vi "host_for_Tx_and_Rx_with scope_scope_cal_file_gen.vi"() -> ()   [LabVIEW 2021]
uses:
  <vilib>/userdefined/High Color/nirio_resource_hc.ctl
  use with scope/states_for scope.ctl
  classes/5785_2_x_1600MHz/5785_2_x_1600MHz.lvclass
  C:/Users/PXIe8108_Demo/Documents/CHAIM DATA/chaim/5785_sync_for_elbit/tx_pulse/pulse Tx Folder_lv_21/EMEA_ADG_EW_Multi_Emitter_Scenarios/classes/device_type/device_type.lvclass
  CTL/user config.ctl
  <instrlib>/niScope/Controls/niScope vertical coupling.ctl
  <instrlib>/niScope/Controls/niScope timestamp type.ctl
  <vilib>/Analysis/1siggen.llb/Ramp Pattern by Delta.vi
  <instrlib>/niScope/Configure/Trigger/niScope Configure Trigger Edge.vi
  <instrlib>/niScope/Acquire/Fetch/niScope Multi Fetch WDT.vi
  <vilib>/Analysis/NI_AALBase.lvlib
  classes/device_type/device_type.lvclass
panel:
  out "run number":i32
  in  "number of runs for cal":dbl=15.0 format="%#_13g"
  in  "read file":bool
  in  "save file":bool=TRUE
  in  "file path":path=path "C:/Users/PXIe8108_Demo/Documents/CHAIM DATA/chaim/5785_sync_for_elbit/tx_pulse/pulse Tx Folder_lv_21/EMEA_ADG_EW_Multi_Emitter_Scenarios/data/scope_cal_file.tdms"
  out "state":T1
  in  "cal":bool=TRUE
  in  "cal mode":bool=TRUE
  out "delta phase(deg)":cluster{"freqency":dbl[], "Array":dbl[]}[](graph)
  out "delta amp (dB)":cluster{"Array":dbl[], "Array":dbl[]}[](graph)
  in  "Channel Name":string="0,3"
  in  "Resource Name":refnum<k15>="scope1" caption="Resource Name(s)"
  in  "pulse amplitude (dB)":dbl=-40.0 format="%#_13g"
  in  "pulse duration (s)":dbl=0.0002 format="%#_13p"
  in  "frequncy comb":cluster{"start":dbl, "end":dbl, "delta":dbl}={"start"=5000000.0, "end"=300000000.0, "delta"=500000.0} {"delta" format="%#_6p"; "end" format="%#_6p"; "start" format="%#_6p"}
  in  "devicess":T2[](array[typedef])=["5785_00", "5785_01", "5785_02"]
  # "5785 system alignment scope cal"
  # "RF setup"
  # "Cal Data"
  # "HW setup"
  # "scope mapping:\nchannel 0 => 5785_02 _0 \nchannel 1 => 5785_01 _0 \nchannel 2 => 5785_01 _1 \nchannel 3 => 5785_00 _1"
  # "Cal test"
  # "SW setup"
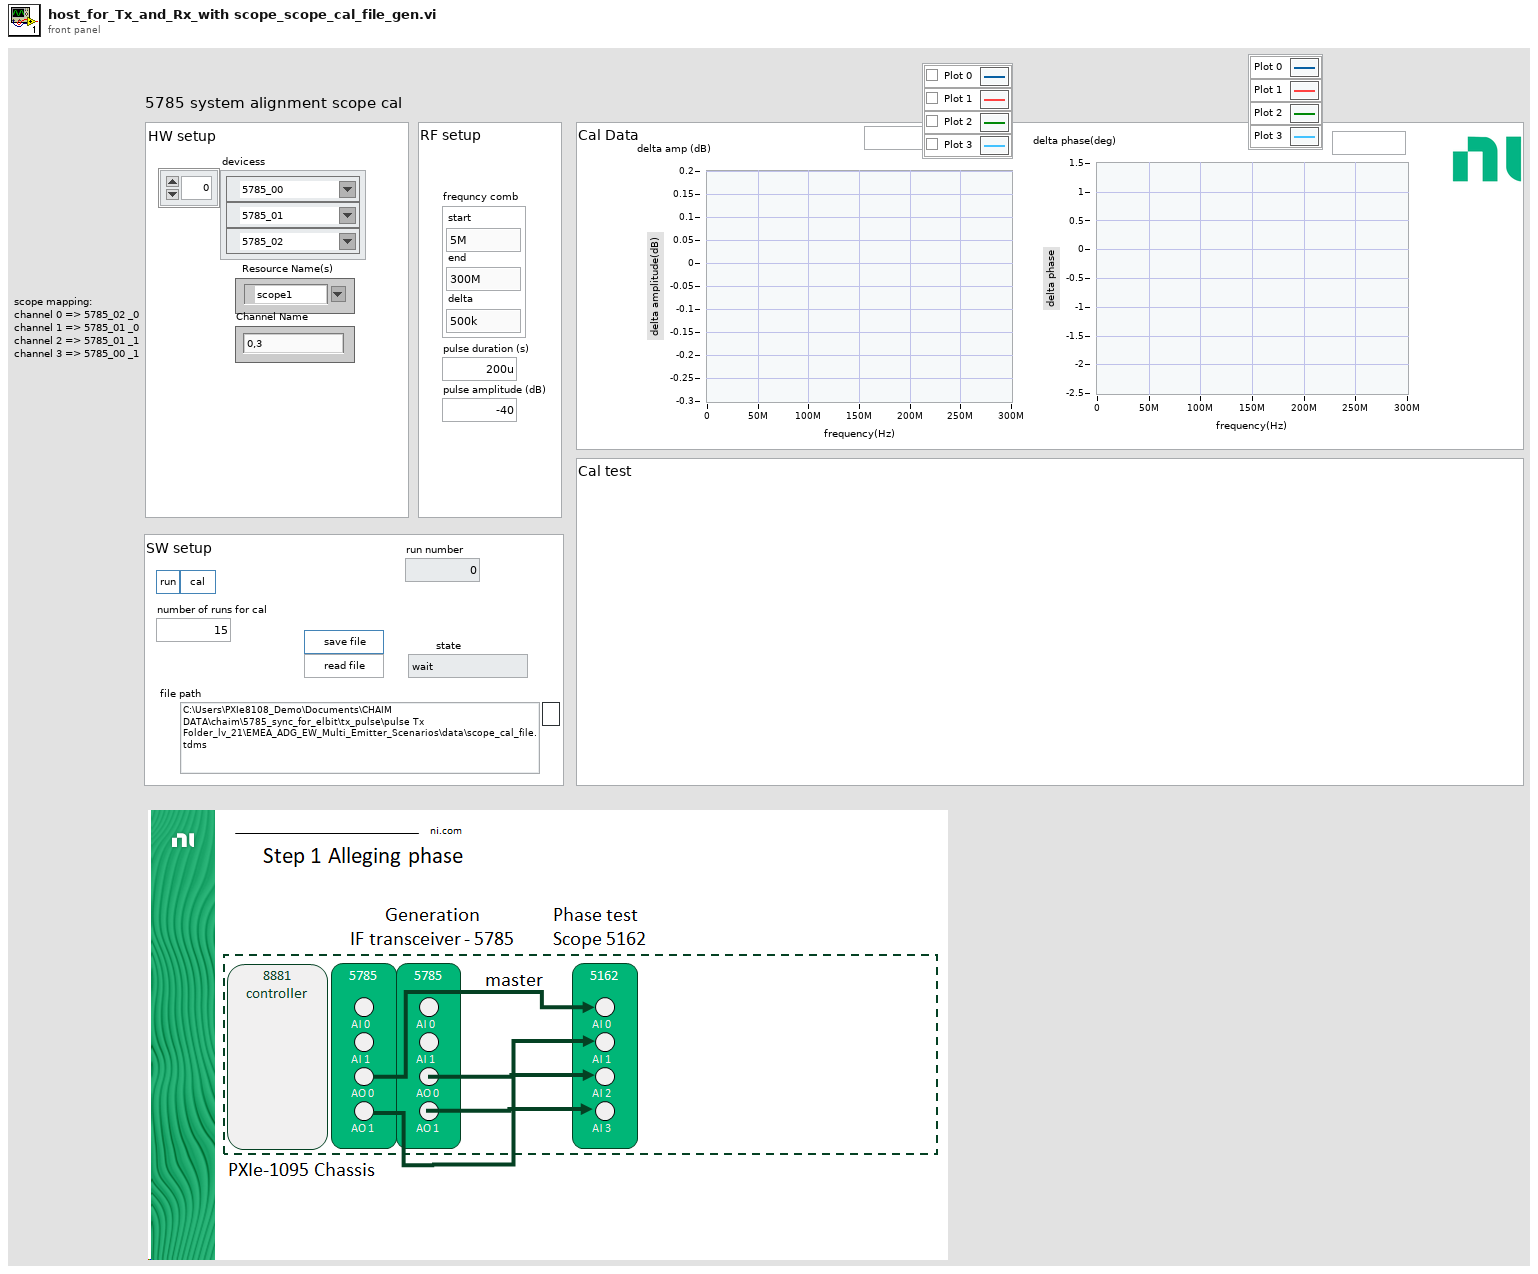
[diagram p1: front panel]
types:
  T1 = typedef "states_for scope.ctl" = enum16{"wait", "update ME config", "gen secenario", "INI ME", "INI scope", "trig", "close ME", "run mesearment", "save cal data", "get file data", "gen PDW file", "keep the data", "reset memory data", "prime the fifo"}
  T2 = typedef "nirio_resource_hc.ctl" = tag
  T3 = cluster{"freqency":dbl[], "phase":dbl[], "amp":dbl[]}[]
  T4 = cluster{"freqency":dbl[], "phase":dbl[], "amp":dbl[]}
  T5 = typedef "user config.ctl" = cluster{"vst_device":refnum<k15>[], "RF gain ":dbl, "buffer size":u32, "center frequency (Hz) ":dbl, "P2P sample rate":dbl, "mode":enum16{"USRP - 180MHz", "5785 - 2*180MHz", "5785 - 3.2GHz", "P2P - VST"}, "devicess":T2[], "gen for df":bool, "Rx settings":cluster{"min PW         ":dbl, "max gap        ":dbl, "detection bar":dbl, "peak detect                        ":bool}, "use arb files":bool}
  T6 = enum16{"open", "open or create", "create or replace", "create", "open (read-only)"}
  T7 = typedef "niScope vertical coupling.ctl" = i32
  T8 = typedef "PDW_lv2.ctl" = cluster{"t start":dbl, "frequency (Hz)":dbl, "duration (sec)":dbl, "mod type":T9, "mod depth":dbl, "phase (rad)":dbl[], "amp (lin)":dbl[]}
  T9 = typedef "mode_type.ctl" = enum8{"CW", "from memory 1", "NC - cw", "LFM", "BPSK", "QPSK"}
  T10 = typedef "niScope timestamp type.ctl" = i32
  T11 = cluster{"frequncy":dbl, "d amp":dbl, "d phase":dbl}[]
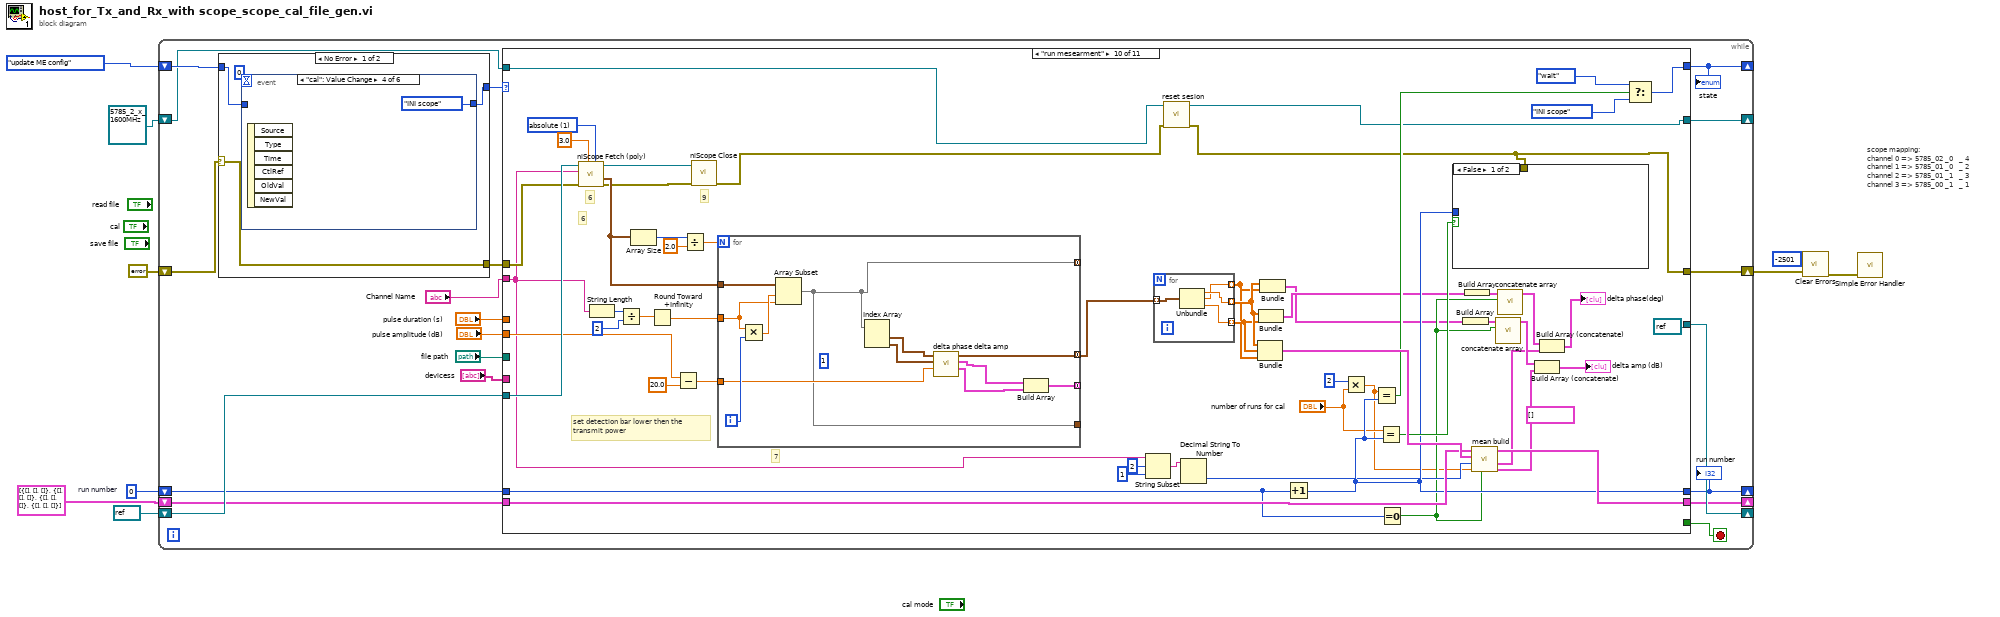
[diagram p0: block diagram]
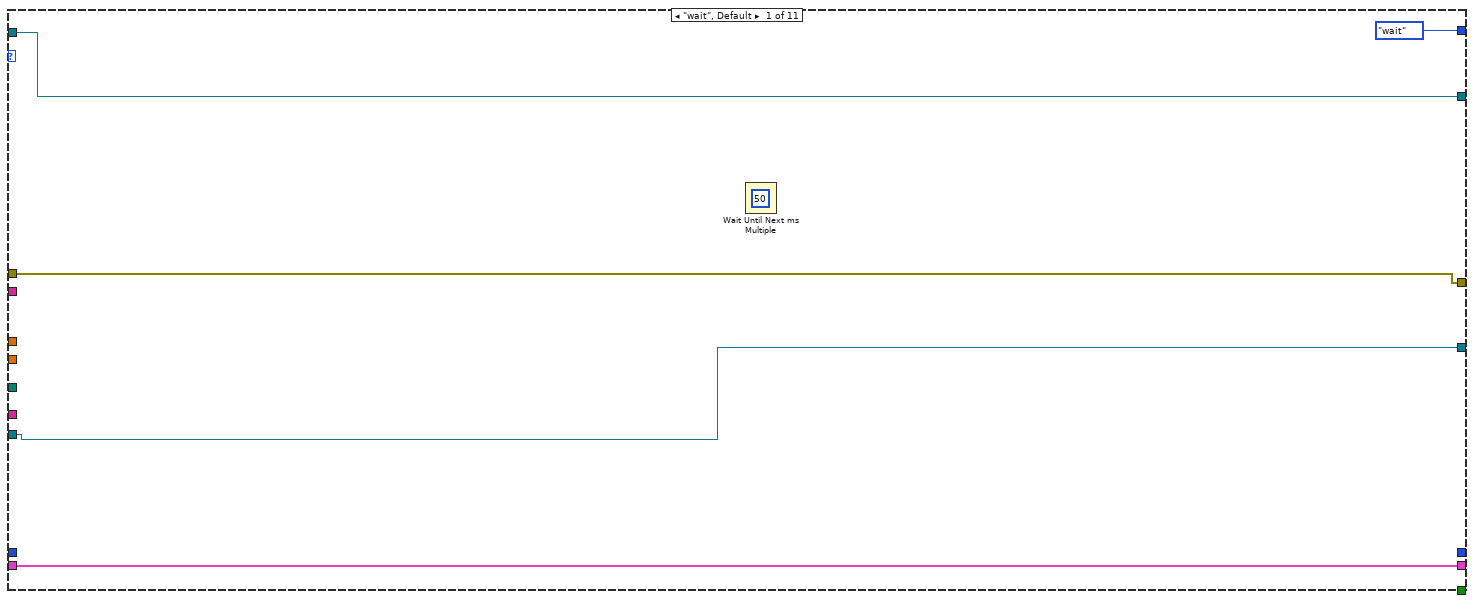
[diagram p2: hidden frame]
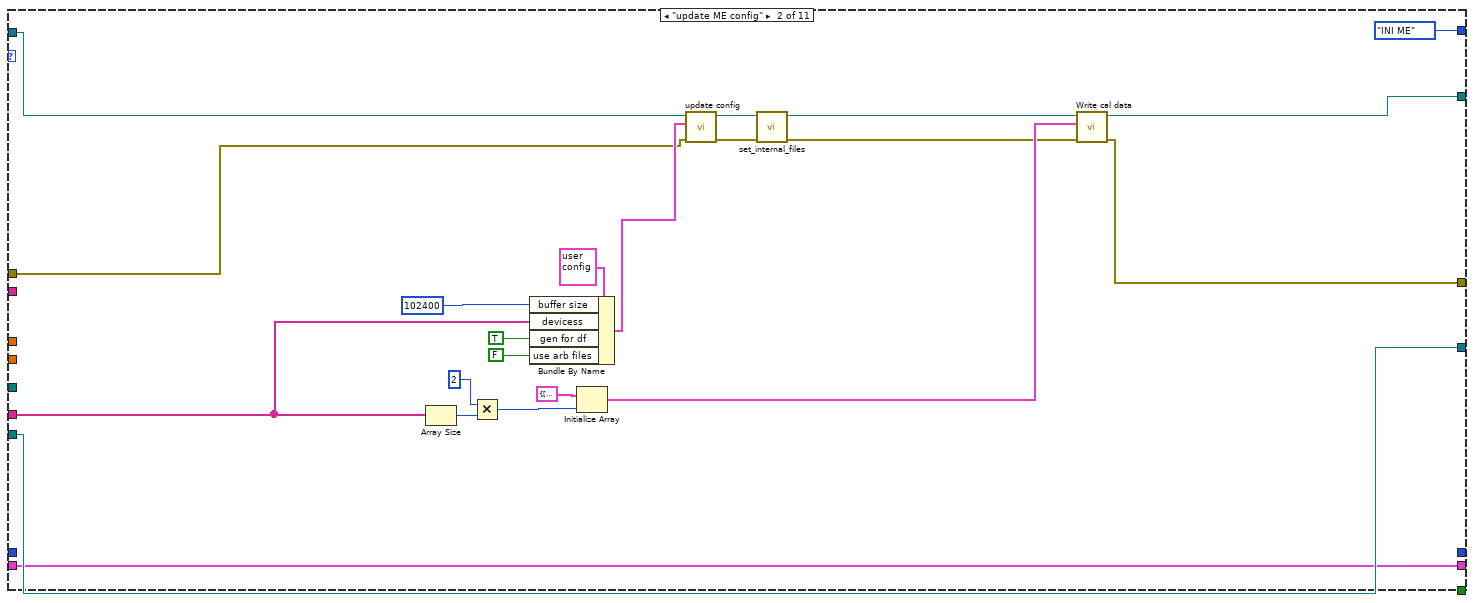
[diagram p3: hidden frame]
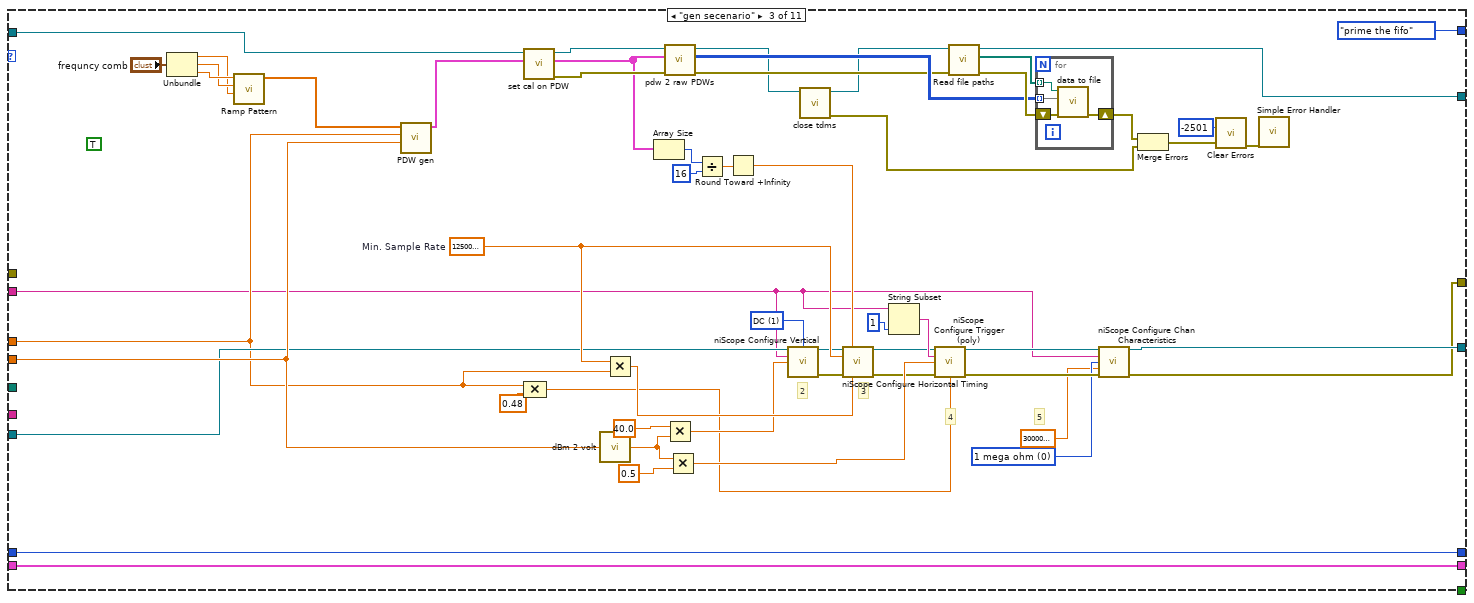
[diagram p4: hidden frame]
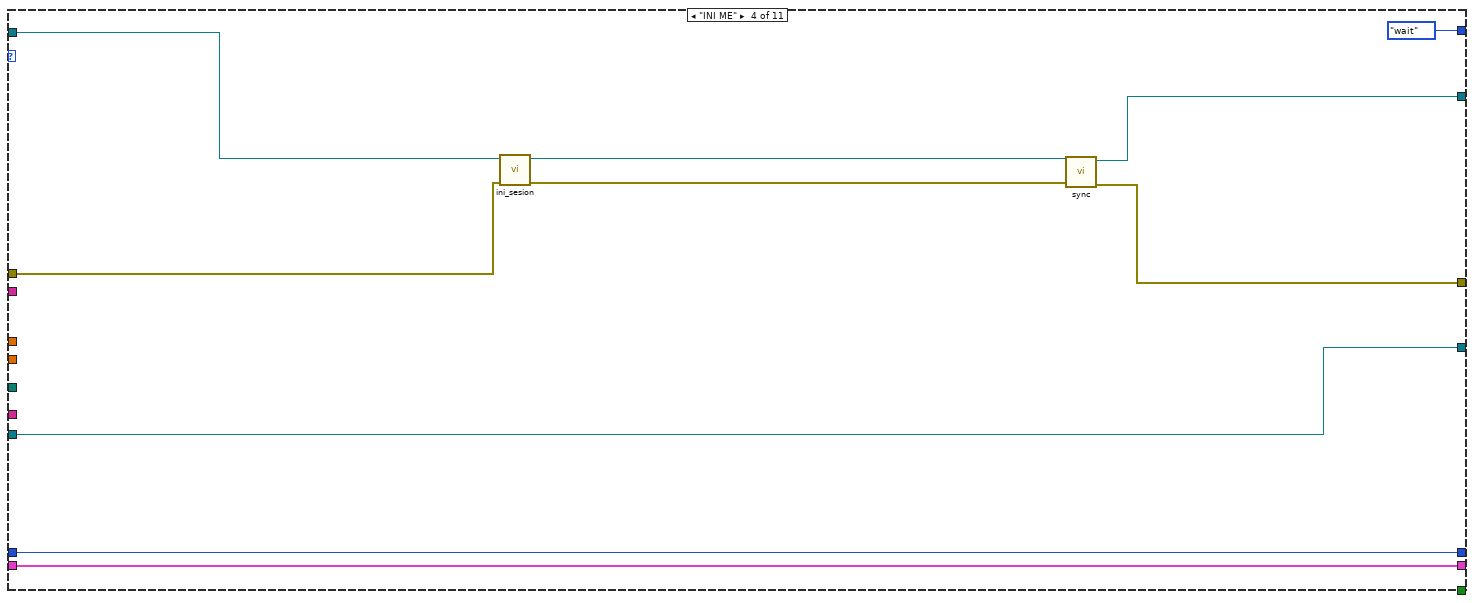
[diagram p5: hidden frame]
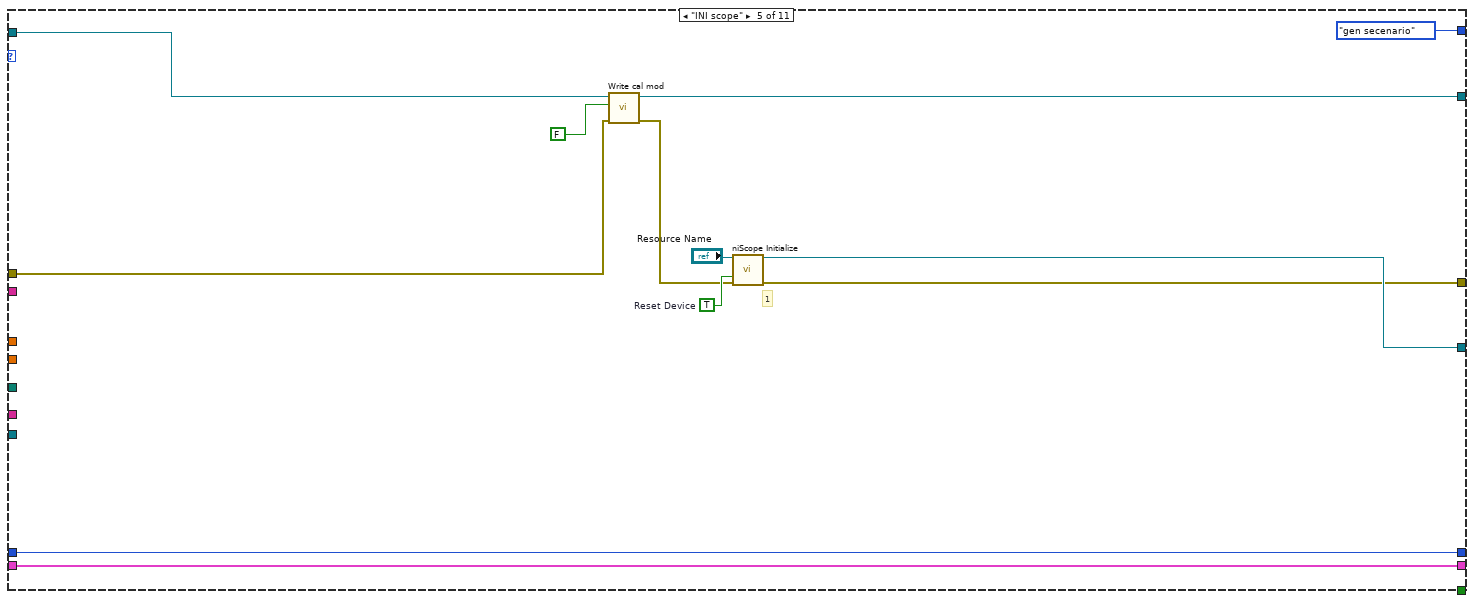
[diagram p6: hidden frame]
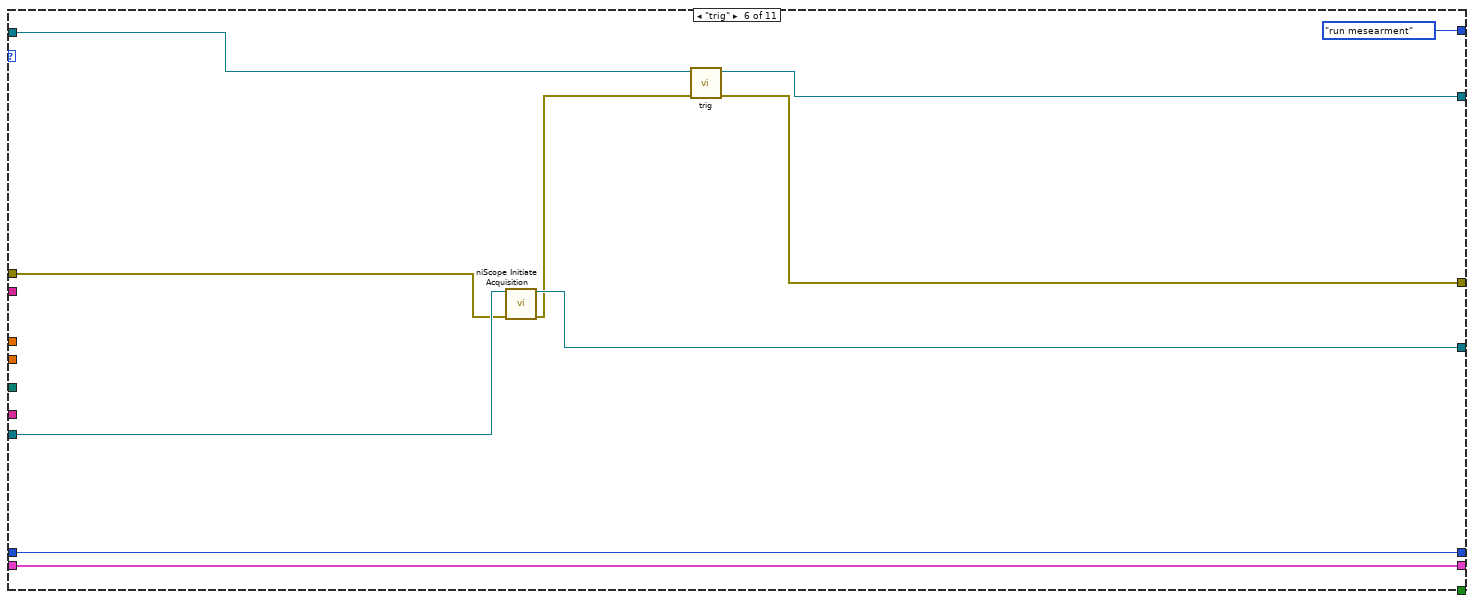
[diagram p7: hidden frame]
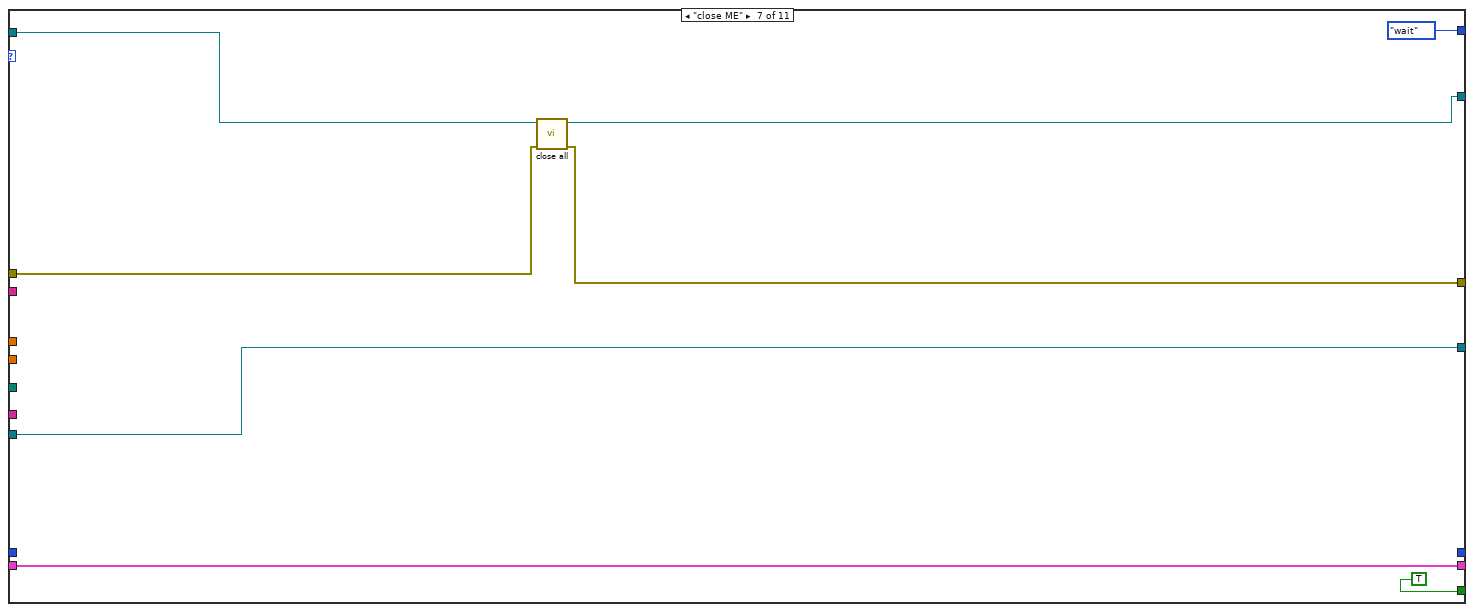
[diagram p8: hidden frame]
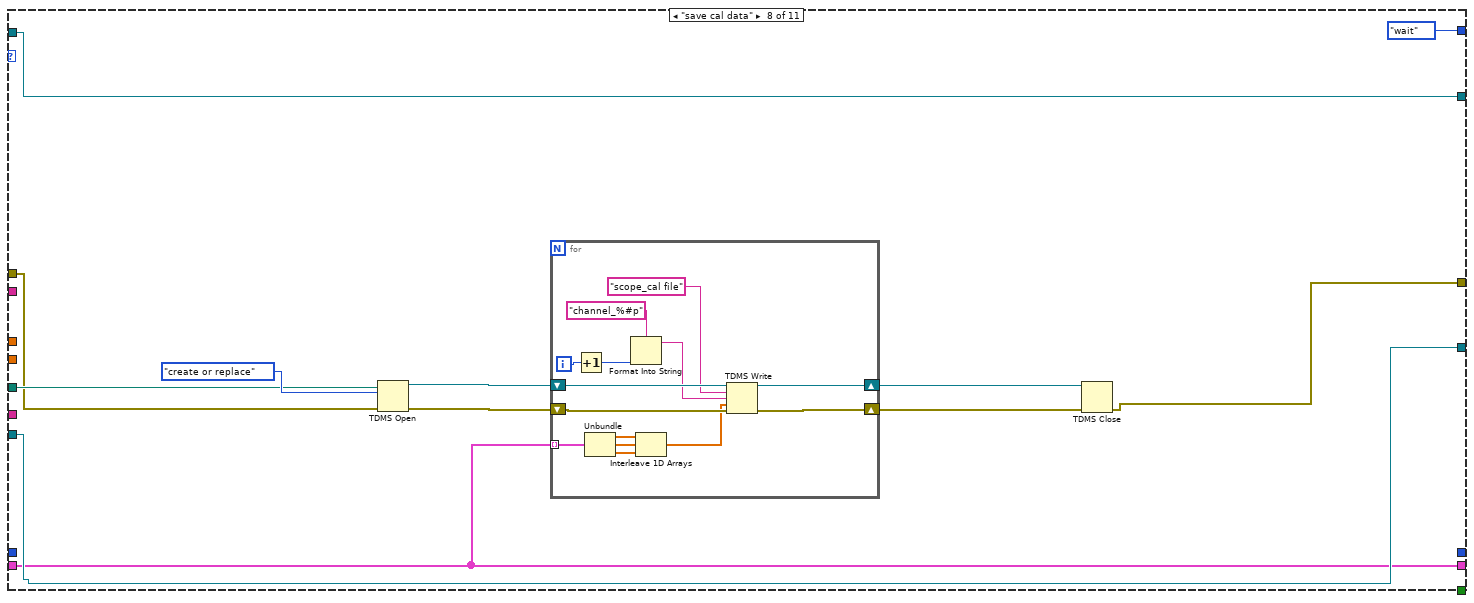
[diagram p9: hidden frame]
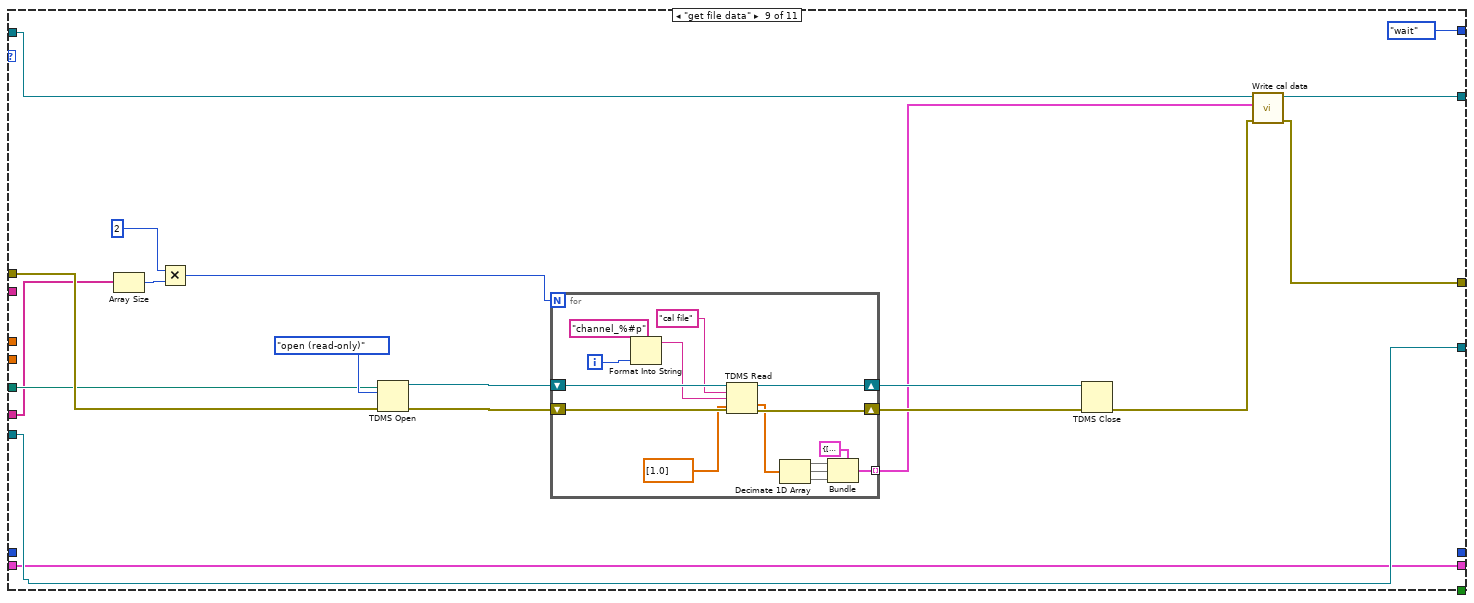
[diagram p10: hidden frame]
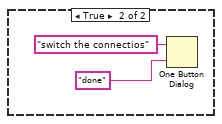
[diagram p11: hidden frame]
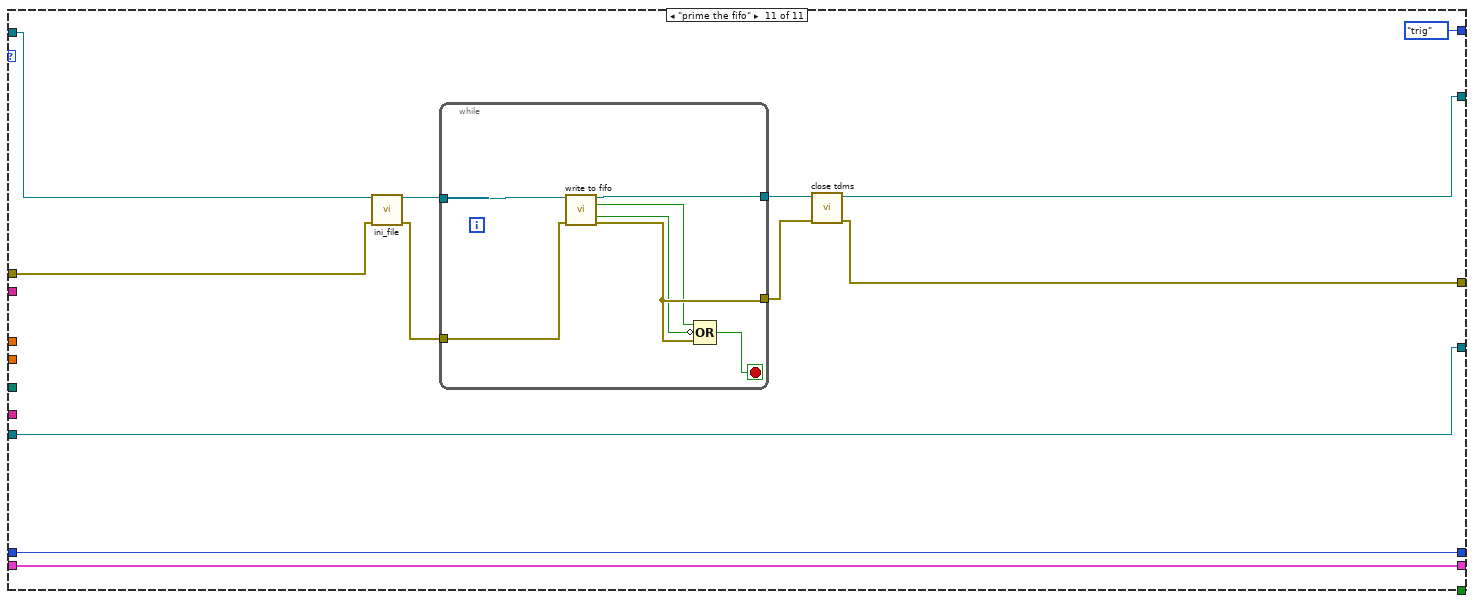
[diagram p12: hidden frame]
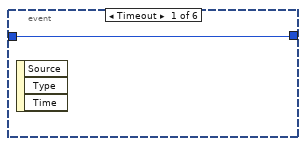
[diagram p13: hidden frame]
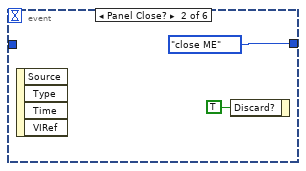
[diagram p14: hidden frame]
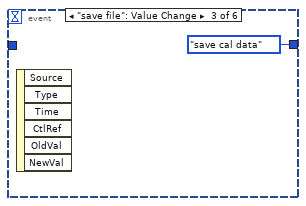
[diagram p15: hidden frame]
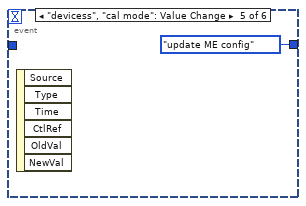
[diagram p16: hidden frame]
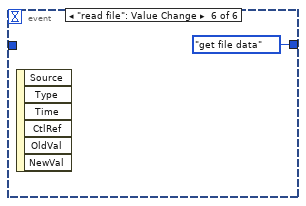
[diagram p17: hidden frame]
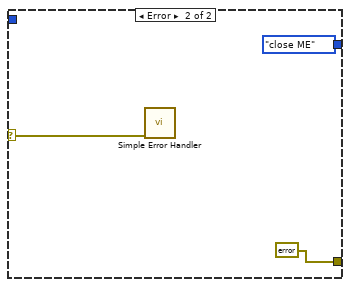
[diagram p18: hidden frame]
diagram:
  (unwired) -2501 ("specific error code to clear (0: all)")
  w4 = 0  # run number
  # "scope mapping:\nchannel 0 => 5785_02 _0   _ 4\nchannel 1 => 5785_01 _0   _ 2 \nchannel 2 => 5785_01 _1   _ 3\nchannel 3 => 5785_00 _1   _ 1"
  n1 = while {
    shift-right: [w15] -> _
    shift-left: states_for_scope."update ME config" -> [w26]
    shift-right: [w23] -> w3
    shift-left: errorcluster {"status"=FALSE, "code"=0, "source"=""} ("error out") -> [w28]
    shift-right: [w20] -> _
    shift-left: refnum<k15> refnum ("instrument handle out") -> [w19]
    shift-right: [w24] -> _
    shift-left: refnum<class "5785_2_x_1600MHz.lvclass"> refnum ("5785_2_x_1600MHz.lvclass") -> [w17]
    shift-right: [w11] -> _
    shift-left: w4 -> [w12]
    shift-right: [w10] -> _
    shift-left: T3 [{"freqency"=[], "phase"=[], "amp"=[]}, {"freqency"=[], "phase"=[], "amp"=[]}, {"freqency"=[], "phase"=[], "amp"=[]}, {"freqency"=[], "phase"=[], "amp"=[]}] ("memory data") -> [w9]
    stop <- w16 stop-if-true
    n2 = case shown="No Error" w28 {
      selector: w28 -> [w311 w321]
      tunnel: [w309 states_for_scope."close ME"] -> w27
      tunnel: w26 -> [w310 _]
      tunnel: [w311 errorcluster {"status"=FALSE, "code"=0, "source"=""} ("error IO")] -> w25
      frame No Error {
        n3 = event shown="[3] \"cal\": Value Change" {
          selector: _ -> [_ _ _ _ _ _]
          dyn-events: _ -> [_ _ _ _ _ _]
          timeout: 0 -> [_ _ _ _ _ _]
          tunnel: w310 -> [w312 _ _ _ _ _]
          tunnel: [w312 states_for_scope."close ME" states_for_scope."save cal data" states_for_scope."INI scope" states_for_scope."update ME config" states_for_scope."get file data"] -> w309
          event Timeout {
            n4 = event-data() -> ()  [unwired: 1 in, 3 out]
          }
          event Panel Close? {
            n5 = event-data() -> ()  [unwired: 1 in, 4 out]
            n6 = event-data("Discard?"=TRUE) -> ()  [unwired: 1 in, 1 out]
          }
          event "save file": Value Change {
            n7 = event-data() -> ()  [unwired: 1 in, 6 out]
          }
          event "cal": Value Change {
            n8 = event-data() -> ()  [unwired: 1 in, 6 out]
          }
          event "devicess", "cal mode": Value Change {
            n9 = event-data() -> ()  [unwired: 1 in, 6 out]
          }
          event "read file": Value Change {
            n10 = event-data() -> ()  [unwired: 1 in, 6 out]
          }
        }
      }
      frame Error {
        n11 = call <vilib>:"Simple Error Handler.vi"("error in (no error)"=w321) -> ()  [unwired: 4 in, 5 out]
      }
    }
    n12 = case shown="\"run mesearment\"" w27 {
      tunnel: w25 -> [w32 w43 _ w122 w128 w145 w153 w157 w197 w259 w293]
      tunnel: [w33 w40 w82 w117 w132 w141 w154 w158 w186 w218 w291] -> w24
      tunnel: [w32 w39 w66 w116 w134 w138 w152 w161 w183 w216 w292] -> w23
      tunnel: "pulse duration (s)" -> [_ _ w83 _ _ _ _ _ _ _ _]
      tunnel: "pulse amplitude (dB)" -> [_ _ w85 _ _ _ _ _ _ w256 _]
      tunnel: [w31 w46 w67 w121 w135 w146 w151 w166 w199 refnum<k15> refnum ("instrument handle out") w290] -> w20
      tunnel: w19 -> [w31 w46 w84 w121 _ w147 w151 w166 w199 w260 w290]
      tunnel: "Channel Name" -> [_ _ w63 _ _ _ _ _ _ w236 _]
      tunnel: w17 -> [w33 w36 w74 w123 w129 w140 w155 w158 w187 w219 w294]
      tunnel: [_ _ _ _ _ _ TRUE _ _ _ _] -> w16
      tunnel: [states_for_scope."wait" states_for_scope."INI ME" states_for_scope."prime the fifo" states_for_scope."wait" states_for_scope."gen secenario" states_for_scope."run mesearment" states_for_scope."wait" states_for_scope."wait" states_for_scope."wait" w243 states_for_scope."trig"] -> w15
      tunnel: "file path" -> [_ _ _ _ _ _ _ w159 w192 _ _]
      tunnel: "devicess" -> [_ w42 _ _ _ _ _ _ w189 _ _]
      tunnel: w12 -> [_ _ w71 w119 w130 w143 _ _ _ w249 w295]
      tunnel: [_ _ w71 w119 w130 w143 _ _ _ w247 w295] -> w11
      tunnel: [w29 w35 w57 w118 w126 w142 w148 w156 w182 w251 w296] -> w10
      tunnel: w9 -> [w29 w35 w57 w118 w126 w142 w148 w156 w182 w250 w296]
      frame "wait", Default {
        n13 = Wait Until Next ms Multiple(millisecond multiple=u32 50) -> ()  [unwired: 1 out]
      }
      frame "update ME config" {
        n14 = Array Size(array=w42) -> (size(s)=w49:i32)
        n15 = Multiply(x=2, y=w49) -> (x*y=w47:i32)
        n16 = Bundle By Name(cluster=T5 {"vst_device"=["VST_1", "VST_2"], "RF gain "=10.0, "buffer size"=524288, "center frequency (Hz) "=1000000000.0, "P2P sample rate"=200000000.0, "mode"=enum."5785 - 2*180MHz", "devicess"=["IF_transiver_0", "IF_transiver_1", "IF_transiver_2"], "gen for df"=FALSE, "Rx settings"={"min PW         "=0.0, "max gap        "=0.0, "detection bar"=0.0, "peak detect                        "=FALSE}, "use arb files"=TRUE} ("user configurations"), "buffer size"=u32 102400, "devicess"=w42, "gen for df"=TRUE, "use arb files"=FALSE) -> (w56:T5)
        n17 = Initialize Array(T4 {"freqency"=[], "phase"=[], "amp"=[]}, w47) -> (w41:T3)
        n18 = call-dynamic "update config.vi"("error in (no error)"=w43, "user configurations"=w56, "5785_2_x_1600MHz in"=w36) -> ("error out"=w54:errorcluster, "5785_2_x_1600MHz out"=w55:refnum<class "5785_2_x_1600MHz.lvclass">)  [unwired: 5 in, 2 out]
        n19 = call-dynamic "set_internal_files.vi"("error in (no error)"=w54, "device_type in"=w55) -> ("error out"=w37:errorcluster, "device_type out"=w38:refnum<class "5785_2_x_1600MHz.lvclass">)  [unwired: 8 in]
        n20 = call-dynamic "Write cal data.vi"("error in (no error)"=w37, "cal data"=w41, "device_type in"=w38) -> ("error out"=w39:errorcluster, "device_type out"=w40:refnum<class "5785_2_x_1600MHz.lvclass">)  [unwired: 7 in]
      }
      frame "gen secenario" {
        w65 = u32 0 items=["1 mega ohm"=0, "50 ohms"=2] ("input impedance")
        w70 = T7 1 items=["AC", "DC", "Ground"] ("vertical coupling")
        (unwired) TRUE ("done")
        w91 = 1250000000.0  # Min. Sample Rate
        # "5"
        # "4"
        # "3"
        # "2"
        n21 = Unbundle("frequncy comb") -> ("start"=w106:dbl, "end"=w107:dbl, "delta"=w108:dbl)
        n22 = call-poly <vilib>:"Ramp Pattern.vi"("start"=w106, "end"=w107, "delta"=w108) -> ("Ramp Pattern"=w109:dbl[])  [unwired: 6 in, 2 out]
        n23 = call "PDW gen.vi"("pulse amplitude"=w85, "pulse duration"=w83, "frequency list"=w109) -> ("PDW out"=w73:T8[])  [unwired: 8 in]
        n24 = call "set cal on PDW.vi"("PDW in"=w73, "device_type in"=w74) -> ("error out"=w75:errorcluster, "cal PDW"=w72:T8[], "device_type out"=w76:refnum<class "5785_2_x_1600MHz.lvclass">)  [unwired: 7 in]
        n25 = Compound Arithmetic op=MULTIPLY(w83, 0.48 ("value")) -> (w95:dbl)
        n26 = call "dBm 2 volt.vi"("dBm"=w85) -> ("V"=w96:dbl)
        n27 = Multiply(x=w91, y=w83) -> (x*y=w99:dbl)
        n28 = Array Size(array=w72) -> (size(s)=w110:i32)
        n29 = call-dynamic "pdw 2 raw PDWs.vi"("error in (no error)"=w75, "PDWs"=w72, "device_type in"=w76) -> ("error out"=w101:errorcluster, "Array"=w103:u64[][], "device_type out"=w78:refnum<class "5785_2_x_1600MHz.lvclass">)  [unwired: 6 in]
        n30 = Multiply(x=40.0, y=w96) -> (x*y=w98:dbl)
        n31 = Multiply(x=w96, y=0.5) -> (x*y=w97:dbl)
        n32 = Divide(x=w110, y=16) -> (x/y=w111:dbl)
        n33 = Round Toward +Infinity(x=w111) -> (ceil(x): smallest int >= x=w86:dbl)
        n34 = call <instrlib>:"niScope Configure Vertical.vi"("instrument handle"=w84, "vertical coupling"=w70, "channels"=w63, "vertical range"=w98) -> ("instrument handle out"=w80:refnum<k15>, "error out"=w79:errorcluster)  [unwired: 10 in]
        n35 = call-dynamic "close tdms.vi"("device_type in"=w78) -> ("error out"=w60:errorcluster, "device_type out"=w77:refnum<class "5785_2_x_1600MHz.lvclass">)  [unwired: 9 in]
        n36 = call <instrlib>:"niScope Configure Horizontal Timing.vi"("instrument handle"=w80, "number of records"=w86, "min sample rate"=w91, "error in"=w79, "min record length"=w99) -> ("instrument handle out"=w93:refnum<k15>, "error out"=w92:errorcluster)  [unwired: 9 in]
        n37 = String Subset(string=w63, length (rest)=1 ("length (rest)")) -> (substring=w94:string)  [unwired: 1 in]
        n38 = call-poly <instrlib>:"niScope Configure Trigger (poly).vi"("instrument handle"=w93, "trigger source"=w94, "trigger level"=w97, "error in"=w92, "trigger delay"=w95) -> ("instrument handle out"=w69:refnum<k15>, "error out"=w68:errorcluster)  [unwired: 9 in]
        n39 = call-dynamic "Read file paths.vi"("error in (no error)"=w101, "device_type in"=w77) -> ("error out"=w104:errorcluster, "file paths"=w102:path[], "device_type out"=w82:refnum<class "5785_2_x_1600MHz.lvclass">)  [unwired: 6 in, 1 out]
        n40 = for {
          tunnel: w103 -> [w113] mode=indexing
          shift-right: [w114] -> w61
          shift-left: w104 -> [w115]
          tunnel: w102 -> [w112] mode=indexing
          n41 = call "data to file.vi"("error in (no error)"=w115, "Array"=w113, "Path"=w112) -> ("error out"=w114:errorcluster)  [unwired: 8 in]
        }
        n42 = call <instrlib>:"niScope Configure Chan Characteristics.vi"("instrument handle"=w69, "channels"=w63, "input impedance"=w65, "maximum input frequency"=300000000.0, "error in"=w68) -> ("instrument handle out"=w67:refnum<k15>, "error out"=w66:errorcluster)  [unwired: 9 in]
        n43 = Merge Errors(w61, w60) -> (w59:errorcluster)
        n44 = call <vilib>:"Clear Errors.vi"("error in (no error)"=w59, "specific error code to clear (0: all)"=-2501) -> ("error out"=w58:errorcluster)  [unwired: 4 in, 1 out]
        n45 = call <vilib>:"Simple Error Handler.vi"("error in (no error)"=w58) -> ()  [unwired: 4 in, 5 out]
      }
      frame "INI ME" {
        n46 = call-dynamic "ini_sesion.vi"("error in (no error)"=w122, "5785_2_x_1600MHz in"=w123) -> ("error out"=w125:errorcluster, "5785_2_x_1600MHz out"=w124:refnum<class "5785_2_x_1600MHz.lvclass">)  [unwired: 8 in]
        n47 = call-dynamic "sync.vi"("error in (no error)"=w125, "5785_2_x_1600MHz in"=w124) -> ("error out"=w116:errorcluster, "5785_2_x_1600MHz out"=w117:refnum<class "5785_2_x_1600MHz.lvclass">)  [unwired: 8 in]
      }
      frame "INI scope" {
        w136 = TRUE  # Reset Device
        # "1"
        n48 = call-dynamic "Write cal mod.vi"("error in (no error)"=w128, "apply cal data"=FALSE, "device_type in"=w129) -> ("error out"=w131:errorcluster, "device_type out"=w132:refnum<class "5785_2_x_1600MHz.lvclass">)  [unwired: 7 in]
        n49 = call <instrlib>:"niScope Initialize.vi"("resource name"="Resource Name", "reset device"=w136, "error in"=w131) -> ("instrument handle"=w135:refnum<k15>, "error out"=w134:errorcluster)  [unwired: 11 in]
      }
      frame "trig" {
        n50 = call <instrlib>:"niScope Initiate Acquisition.vi"("instrument handle"=w147, "error in"=w145) -> ("instrument handle out"=w146:refnum<k15>, "error out"=w139:errorcluster)  [unwired: 12 in]
        n51 = call-dynamic "trig.vi"("error in (no error)"=w139, "5785_2_x_1600MHz in"=w140) -> ("error out"=w138:errorcluster, "5785_2_x_1600MHz out"=w141:refnum<class "5785_2_x_1600MHz.lvclass">)  [unwired: 8 in]
      }
      frame "close ME" {
        n52 = call-dynamic "close all.vi"("error in (no error)"=w153, "5785_2_x_1600MHz in"=w155) -> ("error out"=w152:errorcluster, "5785_2_x_1600MHz out"=w154:refnum<class "5785_2_x_1600MHz.lvclass">)  [unwired: 8 in]
      }
      frame "save cal data" {
        n53 = TDMS Open(8:w157, 10:T6."create or replace" ("operation (0:open)"), 11:w159) -> (0:w164:errorcluster, 3:w165:refnum<k34>)  [unwired: 4 in]
        n54 = for {
          shift-right: [w179] -> w163
          shift-left: w165 -> [w181]
          shift-right: [w178] -> w162
          shift-left: w164 -> [w180]
          tunnel: w156 -> [w173] mode=indexing
          i -> [w169]
          n55 = Increment(x=w169) -> (x+1=w168:i32)
          n56 = Unbundle(w173) -> ("freqency"=w172:dbl[], "phase"=w171:dbl[], "amp"=w170:dbl[])
          n57 = Format Into String(format string="channel_%#p", w168) -> (resulting string=w175:string)  [unwired: 2 in, 1 out]
          n58 = Interleave 1D Arrays(w172, w171, w170) -> (w177:dbl[])
          n59 = TDMS Write(0:w181, 5:"scope_cal file" ("group name in (Untitled)"), 7:w175, 9:w177, 11:w180) -> (4:w179:refnum<k34>, 15:w178:errorcluster)  [unwired: 1 in, 2 out]
        }
        n60 = TDMS Close(8:w162, 11:w163) -> (0:w161:errorcluster)  [unwired: 1 out]
      }
      frame "get file data" {
        n61 = Array Size(array=w189) -> (size(s)=w191:i32)
        n62 = Multiply(x=2, y=w191) -> (x*y=w188:i32)
        n63 = TDMS Open(8:w197, 10:T6."open (read-only)" ("operation (0:open)"), 11:w192) -> (0:w196:errorcluster, 3:w198:refnum<k34>)  [unwired: 4 in]
        n64 = for {
          N: w188 -> [_]
          shift-right: [w213] -> w195
          shift-left: w198 -> [w215]
          shift-right: [w212] -> w194
          shift-left: w196 -> [w214]
          tunnel: [w201] -> w185 mode=indexing
          i -> [w211]
          n65 = Format Into String(format string="channel_%#p", w211) -> (resulting string=w209:string)  [unwired: 2 in, 1 out]
          n66 = TDMS Read(0:w215, 5:"cal file" ("group name in (Untitled)"), 7:w209, 11:w214, 12:dbl[] [1.0] ("interleaved array")) -> (4:w213:refnum<k34>, 10:w206:dbl[], 15:w212:errorcluster)  [unwired: 3 in, 3 out]
          n67 = Decimate 1D Array(w206) -> (w204:dbl[], w203:dbl[], w202:dbl[])
          n68 = Bundle(cluster=T4 {"freqency"=[], "phase"=[], "amp"=[]}, "freqency"=w204, "phase"=w203, "amp"=w202) -> (w201:T4)
        }
        n69 = TDMS Close(8:w194, 11:w195) -> (0:w184:errorcluster)  [unwired: 1 out]
        n70 = call-dynamic "Write cal data.vi"("error in (no error)"=w184, "cal data"=w185, "device_type in"=w187) -> ("error out"=w183:errorcluster, "device_type out"=w186:refnum<class "5785_2_x_1600MHz.lvclass">)  [unwired: 7 in]
      }
      frame "run mesearment" {
        w233 = T10 1 items=["relative", "absolute"] ("timestamp Type")
        (unwired) T3 [] ("memory data")
        # "set detection bar lower then the\ntransmit power"
        # "6"
        # "9"
        # "7"
        # "6"
        n71 = call-poly <instrlib>:"niScope Fetch (poly).vi"("timestamp Type"=w233, "timeout"=3.0, "error in"=w259, "channels"=w236, "instrument handle"=w260) -> ("error out"=w265:errorcluster, "wfm"=w269:waveform(dbl)[], "instrument handle out"=w264:refnum<k15>)  [unwired: 3 in, 1 out]
        n72 = String Length(string=w236) -> (length=w238:i32)
        n73 = Divide(x=w238, y=2) -> (x/y=w237:dbl)
        n74 = Array Size(array=w269) -> (size(s)=w266:i32)
        n75 = Round Toward +Infinity(x=w237) -> (ceil(x): smallest int >= x=w234:dbl)
        n76 = Subtract(x=w256, y=20.0) -> (x-y=w268:dbl)
        n77 = Divide(x=w266, y=2.0) -> (x/y=w267:dbl)
        n78 = call <instrlib>:"niScope Close.vi"("instrument handle"=w264, "error in"=w265) -> ("error out"=w217:errorcluster)  [unwired: 13 in]
        n79 = for {
          N: w267 -> [_]
          tunnel: w269 -> [w288]
          tunnel: w268 -> [w285]
          tunnel: [w284] -> w270 mode=concatenating
          tunnel: [w278] -> _
          tunnel: w234 -> [w280]
          tunnel: [w278] -> _ mode=concatenating
          tunnel: [w277] -> _ mode=concatenating
          i -> [w287]
          (unwired) 1 ("index")
          n80 = Multiply(x=w280, y=w287) -> (x*y=w286:dbl)
          n81 = Array Subset(array=w288, index=w286, length=w280) -> (w278:waveform(dbl)[])
          n82 = Index Array(array=w278) -> (element #1=w279:waveform(dbl), element #2=w281:waveform(dbl))  [unwired: 2 in]
          n83 = call "delta phase delta amp.vi"("detection bar"=w285, "signal in 2"=w281, "signal in 1"=w279) -> ("PSD 1"=w282:cluster{"f0":dbl, "df":dbl, "magnitude":dbl[]}, "PSD 0"=w283:cluster{"f0":dbl, "df":dbl, "magnitude":dbl[]}, "cal data"=w284:T11)  [unwired: 6 in]
          n84 = Build Array(w283, w282) -> (w277:cluster{"f0":dbl, "df":dbl, "magnitude":dbl[]}[])
        }
        n85 = String Subset(string=w236, offset (0)=2, length (rest)=1 ("length (rest)")) -> (substring=w240:string)
        n86 = for {
          tunnel: w270 -> [w276] mode=indexing
          tunnel: [w275] -> w255 mode=indexing
          tunnel: [w274] -> w254 mode=indexing
          tunnel: [w273] -> w253 mode=indexing
          n87 = Unbundle(w276) -> ("frequncy"=w275:dbl, "d amp"=w273:dbl, "d phase"=w274:dbl)
        }
        n88 = call-dynamic "reset sesion.vi"("error in (no error)"=w217, "5785_2_x_1600MHz in"=w219) -> ("error out"=w216:errorcluster, "5785_2_x_1600MHz out"=w218:refnum<class "5785_2_x_1600MHz.lvclass">)  [unwired: 8 in]
        n89 = Decimal String To Number(string=w240) -> (number=w239:i32)  [unwired: 2 in, 1 out]
        n90 = Bundle(w255, w254, w253) -> (w257:cluster{dbl[], dbl[], dbl[]})  [unwired: 1 in]
        n91 = Bundle(w255, w254) -> (w232:cluster{dbl[], dbl[]})  [unwired: 1 in]
        n92 = Bundle(w255, w253) -> (w228:cluster{dbl[], dbl[]})  [unwired: 1 in]
        n93 = Increment(x=w249) -> (x+1=w247:i32)
        n94 = Multiply(x=2, y="number of runs for cal") -> (x*y=w220:dbl)
        n95 = Equal?(x=w220, y=w247) -> (x = y?=w245:bool)
        n96 = Equal?(x="number of runs for cal", y=w247) -> (x = y?=w252:bool)
        n97 = Equal To 0?(x=w249) -> (x = 0?=w229:bool)
        n98 = case shown="False" w252 {
          tunnel: w247 -> [_ _]
          tunnel: w216 -> [_ _]
          frame False {
          }
          frame True {
            n99 = One Button Dialog(message="switch the connectios", button name ("OK")="done") -> ()  [unwired: 1 out]
          }
        }
        n100 = Build Array(w228) -> (w230:cluster{dbl[], dbl[]}[])
        n101 = Build Array(w232) -> (w231:cluster{dbl[], dbl[]}[])
        n102 = call "mean bulid.vi"("reset data"=w229, "mean factor"=w220, "channel"=w239, "new data"=w257, "memory data"=w250) -> ("amp cal"=w226:cluster{"freqency":dbl[], "Array":dbl[]}, "phase cal"=w224:cluster{"freqency":dbl[], "Array":dbl[]}, "memory data"=w251:T3)  [unwired: 4 in]
        n103 = call "concatenate array.vi"("reset"=w229, "Array"=w230) -> ("appended array"=w227:cluster{"Array":dbl[], "Array":dbl[]}[])  [unwired: 9 in]
        n104 = call "concatenate array.vi"("reset"=w229, "Array"=w231) -> ("appended array"=w223:cluster{"Array":dbl[], "Array":dbl[]}[])  [unwired: 9 in]
        n105 = Build Array (concatenate)(w227, w226) -> (→"delta amp (dB)":cluster{"freqency":dbl[], "Array":dbl[]}[])
        n106 = Build Array (concatenate)(w223, w224) -> (→"delta phase(deg)":cluster{"freqency":dbl[], "Array":dbl[]}[])
        n107 = Select(t=states_for_scope."wait", s=w245, f=states_for_scope."INI scope") -> (s? t:f=w243:T1)
      }
      frame "prime the fifo" {
        n108 = call-dynamic "ini_file.vi"("device_type in"=w294, "error in (no error)"=w293) -> ("device_type out"=w299:refnum<class "5785_2_x_1600MHz.lvclass">, "error out"=w300:errorcluster)  [unwired: 11 in, 1 out]
        n109 = while {
          tunnel: w299 -> [w307]
          tunnel: w300 -> [w306]
          tunnel: [w305] -> w298
          tunnel: [w303] -> w297
          stop <- w304 stop-if-true
          n110 = call-dynamic "write to fifo.vi"("5785_2_x_1600MHz in"=w307, "error in (no error)"=w306) -> ("5785_2_x_1600MHz out"=w305:refnum<class "5785_2_x_1600MHz.lvclass">, "done write file"=w301:bool, "room on fifo"=w302:bool, "error out"=w303:errorcluster)  [unwired: 9 in, 1 out]
          n111 = Compound Arithmetic op=OR(w301, invert w302, w303) -> (w304:bool)
        }
        n112 = call-dynamic "close tdms.vi"("error in (no error)"=w297, "device_type in"=w298) -> ("error out"=w292:errorcluster, "device_type out"=w291:refnum<class "5785_2_x_1600MHz.lvclass">)  [unwired: 8 in]
      }
    }
    "state" <- w15
    "run number" <- w11
  }
  n113 = call <vilib>:"Clear Errors.vi"("error in (no error)"=w3) -> ("error out"=w2:errorcluster)  [unwired: 5 in, 1 out]
  n114 = call <vilib>:"Simple Error Handler.vi"("error in (no error)"=w2) -> ()  [unwired: 4 in, 5 out]
